vi "datatoTIFF.vi"(6 "Image Type":T1=7 items=["Grayscale (U8)", "Grayscale (I16)", "Grayscale (SGL)", "Complex (CSG)", "RGB (U32)", "HSL (U32)", "RGB (U64)", "Grayscale (U16)"], 7 "selected path":path, 10 "filename suffix":string, 11 "Array":u16[][][](array[numeric])) -> ()   [LabVIEW 2015]
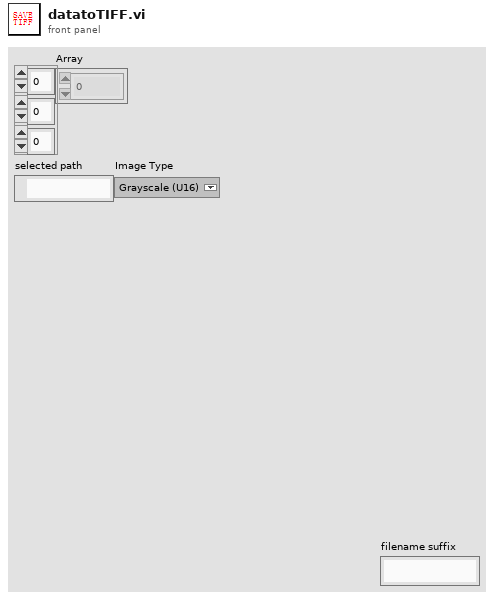
[diagram p1: front panel]
types:
  T1 = typedef "Image Type" = u32
  T2 = typedef "IMAQ Image.ctl" = refnum<image>
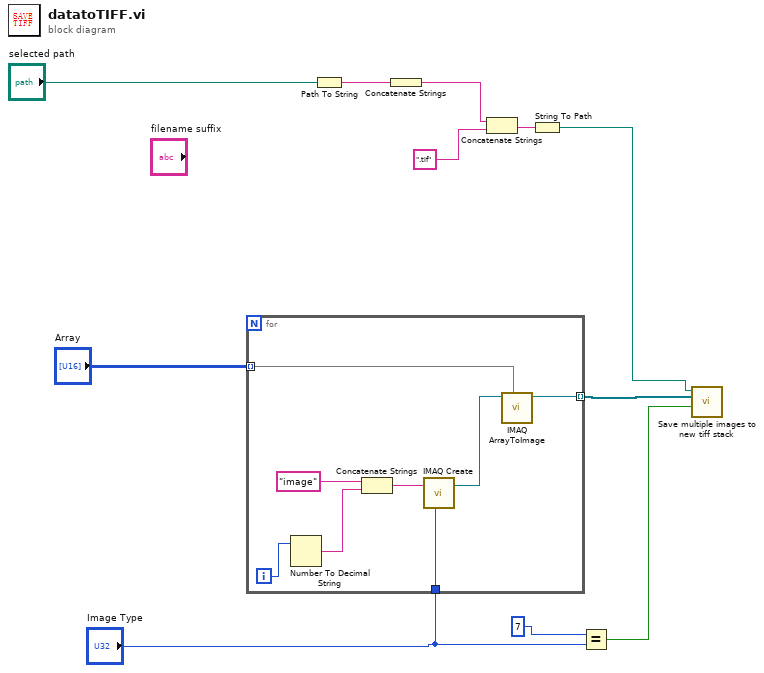
[diagram p0: block diagram]
diagram:
  n1 = for {
    tunnel: "Array" -> [w15] mode=indexing
    tunnel: [w14] -> w5 mode=indexing
    tunnel: "Image Type" -> [w12]
    i -> [w13]
    n2 = Number To Decimal String(number=w13) -> (decimal integer string=w18:string)  [unwired: 1 in]
    n3 = Concatenate Strings("image" ("Image Name"), w18) -> (w17:string)
    n4 = call "IMAQ Create"("Image Name"=w17, "Image Type"=w12) -> ("New Image"=w16:T2)  [unwired: 3 in, 1 out]
    n5 = call "IMAQ ArrayToImage"("Image Pixels (U16)"=w15, "Image"=w16) -> ("Image Out"=w14:T2)  [unwired: 8 in, 1 out]
  }
  n6 = Path To String(path="selected path") -> (string=w10:string)
  n7 = Concatenate Strings(w10) -> (w7:string)
  n8 = Concatenate Strings(w7, ".tif" ("string")) -> (w8:string)
  n9 = String To Path(string=w8) -> (path=w4:path)
  n10 = Equal?(x=7, y="Image Type") -> (x = y?=w1:bool)
  n11 = call "Save multiple images to new tiff stack.vi"(9:w1, "Array of Images (U8, U16, I16)"=w5, "Path"=w4) -> ()  [unwired: 8 in, 1 out]
